vi "m10.wf.ramp.vi"(0 "Waveform In":waveform(dbl), 5 "Ramp Length (s)":dbl, 11 "error in (no error)":errorcluster) -> (4 "Waveform Out":waveform(dbl), 15 "error out":errorcluster)   [LabVIEW 2009]
uses:
  <vilib>/Waveform/WDTOps.llb/WDT Waveform Duration DBL.vi
  <vilib>/measure/NI_MABase.lvlib
  <vilib>/Waveform/WDTOps.llb/WDT Append Waveforms DBL.vi
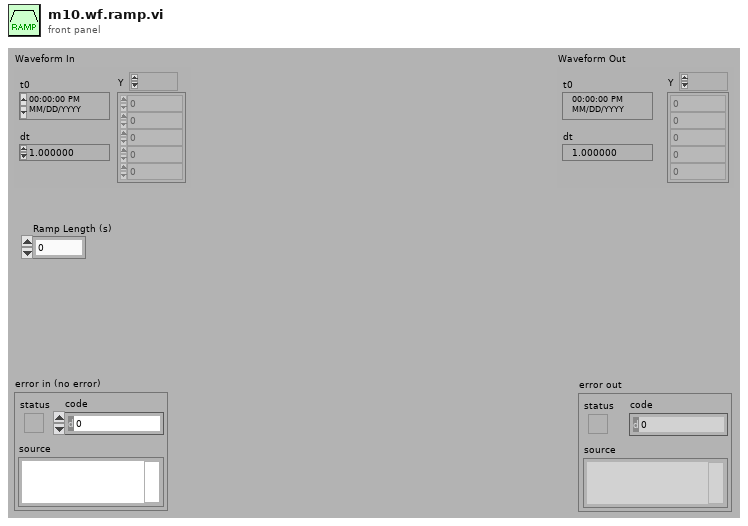
[diagram p1: front panel]
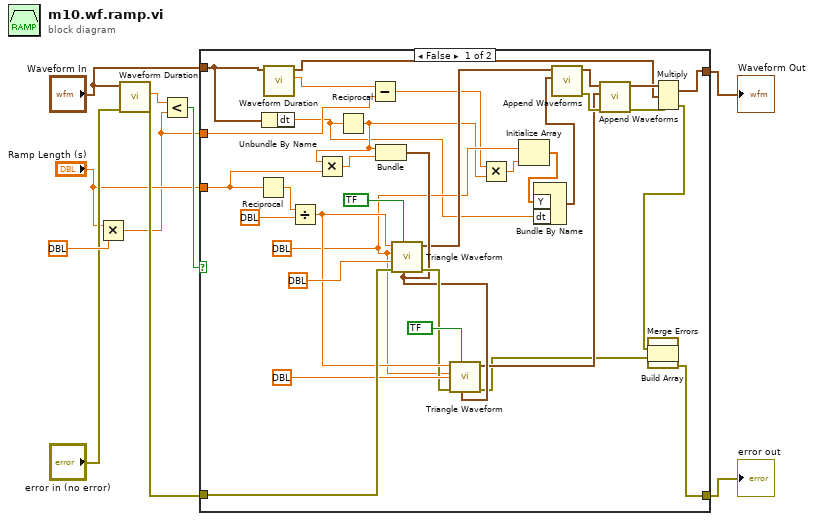
[diagram p0: block diagram]
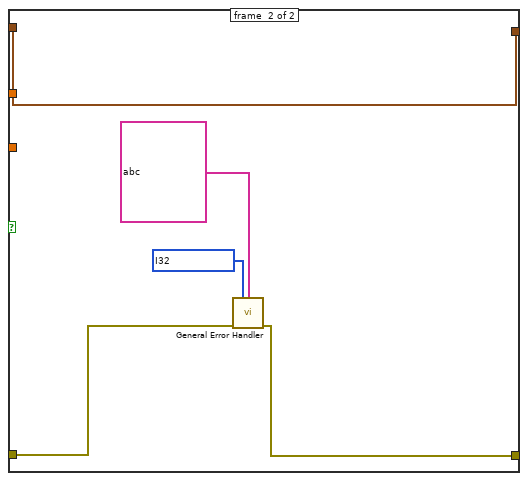
[diagram p2: hidden frame]
diagram:
  n1 = Multiply(x="Ramp Length (s)", y=dbl ?) -> (x*y=w1:dbl)
  n2 = call-poly <vilib>:"Waveform Duration.vi"("error in (no error)"="error in (no error)", "waveform in"="Waveform In") -> ("error out"=w6:errorcluster, "duration"=w10:dbl)  [unwired: 7 in, 1 out]
  n3 = Less?(x=w10, y=w1) -> (x < y?=w8:bool)
  n4 = case shown="False" w8 {
    tunnel: w6 -> [w41 w49]
    tunnel: [w19 w48] -> w3
    tunnel: "Waveform In" -> [w26 w45]
    tunnel: [w23 w45] -> w4
    tunnel: "Ramp Length (s)" -> [w29 _]
    tunnel: w1 -> [w27 _]
    frame #0 {
      w16 = dbl ? ("amplitude")
      n5 = Reciprocal(x=w29) -> (1/x=w44:dbl)
      n6 = Unbundle By Name(w26) -> ("dt"=w13:dbl)
      n7 = call-poly <vilib>:"Waveform Duration.vi"("waveform in"=w26) -> ("duration"=w24:dbl, "waveform out"=w25:waveform(dbl))  [unwired: 8 in, 1 out]
      n8 = Divide(x=w44, y=dbl ?) -> (x/y=w37:dbl)
      n9 = Reciprocal(x=w13) -> (1/x=w14:dbl)
      n10 = Multiply(x=w14, y=w29) -> (x*y=w40:dbl)
      n11 = Subtract(x=w24, y=w27) -> (x-y=w15:dbl)
      n12 = Bundle(w14, w40) -> (w34:cluster{dbl, dbl})  [unwired: 1 in]
      n13 = call <vilib>:"Triangle Waveform.vi"("sampling info"=w34, "reset signal"=bool ?, "error in (no error)"=w41, "phase"=dbl ?, "amplitude"=w16, "frequency"=w37) -> ("error out"=w35:errorcluster, "signal out"=w32:waveform(dbl))  [unwired: 4 in]
      n14 = call <vilib>:"Triangle Waveform.vi"("sampling info"=w34, "reset signal"=bool ?, "error in (no error)"=w35, "phase"=dbl ?, "amplitude"=w16, "frequency"=w37) -> ("error out"=w20:errorcluster, "signal out"=w30:waveform(dbl))  [unwired: 4 in]
      n15 = Multiply(x=w15, y=w14) -> (x*y=w17:dbl)
      n16 = Initialize Array(w16, w17) -> (w18:dbl[])
      n17 = Bundle By Name("Y"=w18, "dt"=w13) -> (w12:waveform(dbl))  [unwired: 1 in]
      n18 = call-poly <vilib>:"Append Waveforms.vi"("waveform B"=w12, "waveform A"=w32) -> ("error out"=w31:errorcluster, "waveform out"=w33:waveform(dbl))  [unwired: 8 in]
      n19 = call-poly <vilib>:"Append Waveforms.vi"("error in (no error)"=w31, "waveform B"=w30, "waveform A"=w33) -> ("error out"=w22:errorcluster, "waveform out"=w28:waveform(dbl))  [unwired: 7 in]
      n20 = Multiply(1:w25, 2:w28, 4:w22) -> (0:w23:waveform(dbl), 3:w21:errorcluster)
      n21 = Build Array(w21, w20) -> (w11:errorcluster[])
      n22 = call <vilib>:"Merge Errors.vi"("error array in"=w11) -> ("error out"=w19:errorcluster)  [unwired: 6 in]
    }
    frame #1 {
      n23 = call <vilib>:"General Error Handler.vi"("[user-defined codes]"=i32[] ?, "[user-defined descriptions]"=string[] ?, "error in (no error)"=w49) -> ("error out"=w48:errorcluster)  [unwired: 8 in, 4 out]
    }
  }
  "Waveform Out" <- w4
  "error out" <- w3
